vi "Format into String.vi"() -> ()   [LabVIEW 2015]
panel:
  out "Formatted String":string
  in  "Has a Driving Licence":bool
  in  "Favourite Colour":u32(colorbox)
  in  "Date of Birth":timestamp
  in  "Name":string
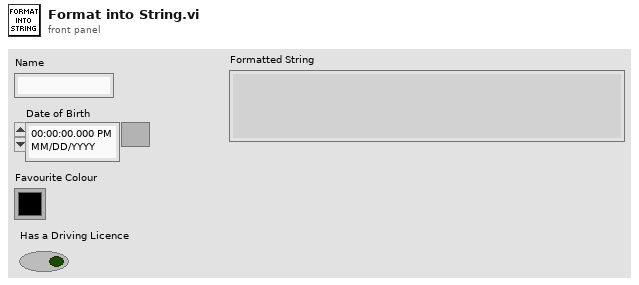
[diagram p1: front panel]
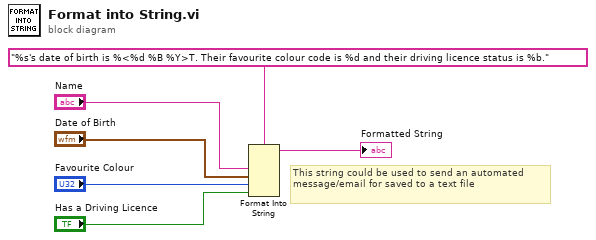
[diagram p0: block diagram]
diagram:
  # "This string could be used to send an automated message/email for saved to a text file"
  n1 = Format Into String(format string="%s's date of birth is %<%d %B %Y>T. Their favourite colour code is %d and their driving licence status is %b.", "Name", "Date of Birth", "Favourite Colour", "Has a Driving Licence") -> (resulting string=→"Formatted String":string)  [unwired: 2 in, 1 out]
